vi "CodigoLabView 2_1.vi"() -> ()   [LabVIEW 2025]
uses:
  <vilib>/Instr/_visa.llb/VISA Configure Serial Port (Instr).vi
panel:
  out "Rele 4":bool
  out "Estado 4":string
  out "Rele 3":bool
  out "Estado 3":string
  out "Rele 2":bool
  out "Estado 2":string
  out "rele 4":string
  in  "Relé N°4":bool
  out "rele 3":string
  in  "Relé N°3":bool
  out "rele 2":string
  in  "Relé N°2":bool
  out "Estado 1":string
  out "rele 1":string
  out "Rele 1":bool
  in  "Relé N°1":bool
  out "Serial Settings":u32
  out "error out 2":errorcluster
  out "Enviando":string
  out "error out":errorcluster
  in  "VISA resource name":refnum<visa-resource-name>
  in  "stop":bool
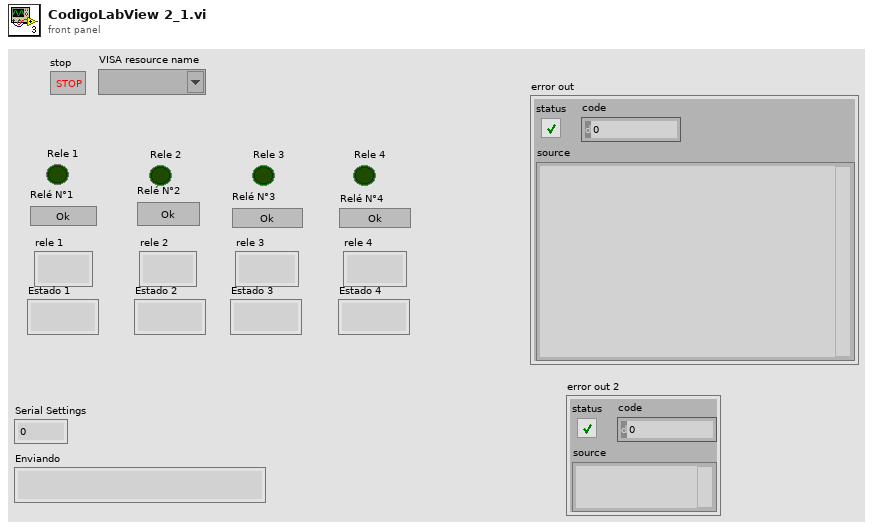
[diagram p1: front panel]
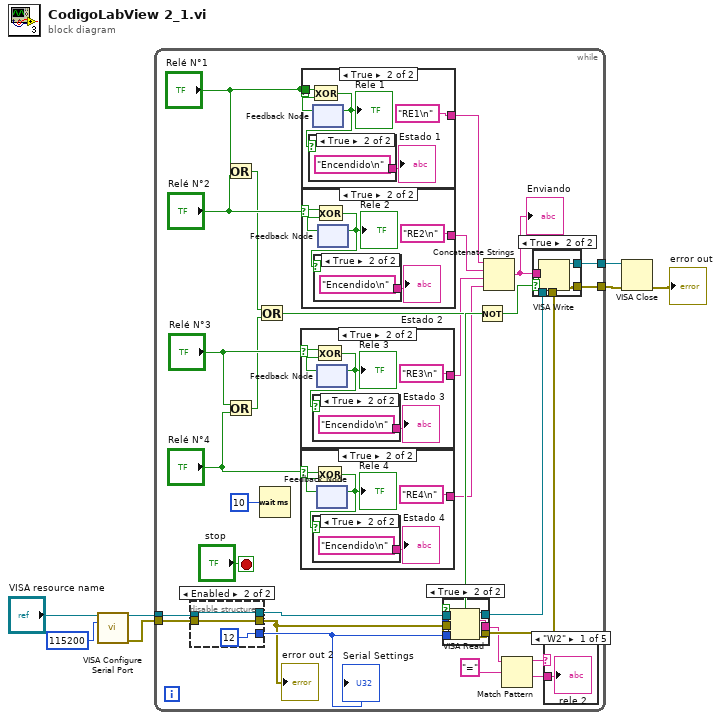
[diagram p0: block diagram]
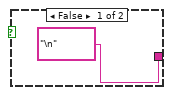
[diagram p2: hidden frame]
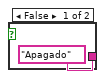
[diagram p3: hidden frame]
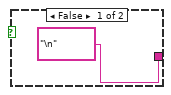
[diagram p4: hidden frame]
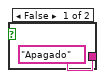
[diagram p5: hidden frame]
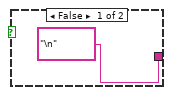
[diagram p6: hidden frame]
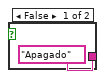
[diagram p7: hidden frame]
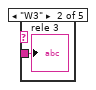
[diagram p8: hidden frame]
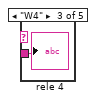
[diagram p9: hidden frame]
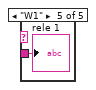
[diagram p11: hidden frame]
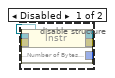
[diagram p12: hidden frame]
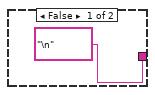
[diagram p15: hidden frame]
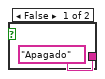
[diagram p16: hidden frame]
diagram:
  n1 = call-poly "VISA Configure Serial Port"("VISA resource name"="VISA resource name", "baud rate (9600)"=u32 115200) -> ("VISA resource name out"=w7:refnum<visa-resource-name>, "error out"=w1:errorcluster)  [unwired: 12 in]
  n2 = while {
    tunnel: w7 -> [w34]
    tunnel: [w32] -> w6
    tunnel: w1 -> [w33]
    tunnel: [w31] -> w5
    stop <- "stop" stop-if-true
    n3 = disable-structure shown="Enabled" {
      disable-tunnel: w34 -> [w68 w71]
      disable-tunnel: w33 -> [w67 w70]
      disable-tunnel: [w66 w71] -> w28
      disable-tunnel: [w65 u32 12 ("Bytes at Port")] -> w27
      disable-tunnel: [w64 w70] -> w26
      frame Disabled {
        n4 = property class="Instr"(reference=w68, error in=w67) -> (reference out=w66:refnum<visa-resource-name>, error out=w64:errorcluster, "Serial Settings:Number of Bytes at Serial Port"=w65:u32)
      }
      frame Enabled {
      }
    }
    "error out 2" <- w26
    "Serial Settings" <- w27
    n5 = Or(x="Relé N°1", y="Relé N°2") -> (x .or. y?=w14:bool)
    n6 = Or(x="Relé N°3", y="Relé N°4") -> (x .or. y?=w13:bool)
    n7 = Or(x=w14, y=w13) -> (x .or. y?=w18:bool)
    n8 = Wait (ms)(milliseconds to wait=u32 10) -> ()  [unwired: 1 out]
    n9 = case shown="True" "Relé N°3" {
      selector: "Relé N°3" -> [_ w45]
      tunnel: ["\n" "RE3\n"] -> w12
      frame False {
      }
      frame True {
        n10 = feedback #1() -> (w48:bool)  [unwired: 1 in]
        n11 = Exclusive Or(1:w48, 2:w45) -> (0:w47:bool)
        "Rele 3" <- w47
        n12 = case shown="True" w47 {
          tunnel: ["Apagado" "Encendido\n"] -> w46
          frame False {
          }
          frame True {
          }
        }
        "Estado 3" <- w46
        n13 = feedback-in #1(w47) -> ()
      }
    }
    n14 = case shown="True" "Relé N°4" {
      selector: "Relé N°4" -> [_ w37]
      tunnel: ["\n" "RE4\n"] -> w11
      frame False {
      }
      frame True {
        n15 = feedback #2() -> (w40:bool)  [unwired: 1 in]
        n16 = Exclusive Or(1:w40, 2:w37) -> (0:w39:bool)
        "Rele 4" <- w39
        n17 = case shown="True" w39 {
          tunnel: ["Apagado" "Encendido\n"] -> w38
          frame False {
          }
          frame True {
          }
        }
        "Estado 4" <- w38
        n18 = feedback-in #2(w39) -> ()
      }
    }
    n19 = case shown="True" "Relé N°1" {
      tunnel: ["\n" "RE1\n"] -> w9
      tunnel: "Relé N°1" -> [_ w91]
      frame False {
      }
      frame True {
        n20 = feedback #3() -> (w90:bool)  [unwired: 1 in]
        n21 = Exclusive Or(1:w90, 2:w91) -> (0:w89:bool)
        "Rele 1" <- w89
        n22 = case shown="True" w89 {
          tunnel: ["Apagado" "Encendido\n"] -> w88
          frame False {
          }
          frame True {
          }
        }
        "Estado 1" <- w88
        n23 = feedback-in #3(w89) -> ()
      }
    }
    n24 = case shown="True" "Relé N°2" {
      selector: "Relé N°2" -> [_ w53]
      tunnel: ["\n" "RE2\n"] -> w10
      frame False {
      }
      frame True {
        n25 = feedback #4() -> (w56:bool)  [unwired: 1 in]
        n26 = Exclusive Or(1:w56, 2:w53) -> (0:w55:bool)
        "Rele 2" <- w55
        n27 = case shown="True" w55 {
          tunnel: ["Apagado" "Encendido\n"] -> w54
          frame False {
          }
          frame True {
          }
        }
        "Estado 2" <- w54
        n28 = feedback-in #4(w55) -> ()
      }
    }
    n29 = Not(x=w18) -> (.not. x?=w25:bool)
    n30 = case shown="True" w25 {
      tunnel: [w73 w79] -> w30
      tunnel: [w72 w78] -> w29
      tunnel: w26 -> [w72 w77]
      tunnel: w28 -> [w73 w76]
      tunnel: w27 -> [_ w75]
      tunnel: [_ w74] -> w23
      frame False {
      }
      frame True {
        n31 = VISA Read(VISA resource name=w76, byte count=w75, error in (no error)=w77) -> (VISA resource name out=w79:refnum<visa-resource-name>, read buffer=w74:string, error out=w78:errorcluster)  [unwired: 1 out]
      }
    }
    n32 = Concatenate Strings(w9, w10, w12, w11) -> (w8:string)
    "Enviando" <- w8
    n33 = Match Pattern(string=w23, regular expression="=") -> (before substring=w21:string, after substring=w20:string)  [unwired: 1 in, 2 out]
    n34 = case shown="True" w18 {
      tunnel: [w81 w86] -> w32
      tunnel: [w80 w85] -> w31
      tunnel: w30 -> [w81 w84]
      tunnel: w29 -> [w80 w83]
      tunnel: w8 -> [_ w82]
      frame False {
      }
      frame True {
        n35 = VISA Write(VISA resource name=w84, write buffer=w82, error in (no error)=w83) -> (VISA resource name out=w86:refnum<visa-resource-name>, error out=w85:errorcluster)  [unwired: 1 out]
      }
    }
    n36 = case shown="\"W2\"" w21 {
      tunnel: w20 -> [w60 w61 w62 _ w63]
      frame "W2" {
        "rele 2" <- w60
      }
      frame "W3" {
        "rele 3" <- w61
      }
      frame "W4" {
        "rele 4" <- w62
      }
      frame "False", Default {
      }
      frame "W1" {
        "rele 1" <- w63
      }
    }
  }
  n37 = VISA Close(VISA resource name=w6, error in (no error)=w5) -> (error out=→"error out":errorcluster)
